vi "AutoFlex.vi"(0 "Inputs":T1={"Slider 1"=0.0, "Slider 2"=-0.007874015748031496}, 1 "Record":bool=TRUE, 2 "Save":bool=TRUE, 3 "Playback":bool, 5 "Delete":bool, 6 "Increase File ID":bool, 7 "Decrease File ID":bool) -> (20 "Outputs":T1={"Slider 1"=0.0, "Slider 2"=-0.007874015748031496}, 22 "File ID":i32)   [LabVIEW 2012]
uses:
  Joystick Event.ctl
panel:
  out "Info Path":path=path "C:/Users/FRC/Desktop/Autoflex/000.txt"
  out "Joystick Event":cluster{"Timestamp":u32, "Input":T1}={"Timestamp"=657367, "Input"={"Slider 1"=0.0, "Slider 2"=-0.007874015748031496}}
  out "Timestamp":u32=657367
  out "Joystick Event Array":cluster{"Timestamp":u32, "Input":T1}[](array[cluster])=[{"Timestamp"=234633, "Input"={"Slider 1"=-0.047244094488188976, "Slider 2"=0.0}}, {"Timestamp"=234778, "Input"={"Slider 1"=-0.08661417322834646, "Slider 2"=-0.06299212598425197}}, {"Timestamp"=234848, "Input"={"Slider 1"=-0.08661417322834646, "Slider 2"=-0.14173228346456693}}, {"Timestamp"=234900, "Input"={"Slider 1"=-0.10236220472440945, "Slider 2"=-0.18110236220472442}}, {"Timestamp"=234954, "Input"={"Slider 1"=-0.12598425196850394, "Slider 2"=-0.28346456692913385}}, {"Timestamp"=235026, "Input"={"Slider 1"=-0.12598425196850394, "Slider 2"=-0.3228346456692913}}, {"Timestamp"=235372, "Input"={"Slider 1"=-0.12598425196850394, "Slider 2"=-0.3464566929133858}}, {"Timestamp"=235433, "Input"={"Slider 1"=0.07874015748031496, "Slider 2"=-0.4015748031496063}}, {"Timestamp"=235492, "Input"={"Slider 1"=-0.16535433070866143, "Slider 2"=-0.44881889763779526}}, {"Timestamp"=235557, "Input"={"Slider 1"=-0.18110236220472442, "Slider 2"=-0.4881889763779528}}, {"Timestamp"=235623, "Input"={"Slider 1"=-0.18110236220472442, "Slider 2"=-0.5039370078740157}}, {"Timestamp"=236417, "Input"={"Slider 1"=-0.18110236220472442, "Slider 2"=-0.30708661417322836}}, {"Timestamp"=236495, "Input"={"Slider 1"=0.0, "Slider 2"=-0.023622047244094488}}, {"Timestamp"=236541, "Input"={"Slider 1"=0.0, "Slider 2"=-0.007874015748031496}}, {"Timestamp"=236695, "Input"={"Slider 1"=0.0, "Slider 2"=0.0}}, {"Timestamp"=236902, "Input"={"Slider 1"=0.0, "Slider 2"=0.031496062992125984}}, {"Timestamp"=236955, "Input"={"Slider 1"=0.03937007874015748, "Slider 2"=0.09448818897637795}}, {"Timestamp"=237014, "Input"={"Slider 1"=0.11811023622047244, "Slider 2"=0.1732283464566929}}, {"Timestamp"=237078, "Input"={"Slider 1"=0.023622047244094488, "Slider 2"=0.2755905511811024}}, {"Timestamp"=237136, "Input"={"Slider 1"=0.0, "Slider 2"=0.3543307086614173}}, {"Timestamp"=237217, "Input"={"Slider 1"=0.0, "Slider 2"=0.4566929133858268}}, {"Timestamp"=237272, "Input"={"Slider 1"=0.0, "Slider 2"=0.5196850393700787}}, {"Timestamp"=237332, "Input"={"Slider 1"=0.0, "Slider 2"=0.5433070866141733}}, {"Timestamp"=237398, "Input"={"Slider 1"=0.0, "Slider 2"=0.5590551181102362}}, {"Timestamp"=237460, "Input"={"Slider 1"=0.0, "Slider 2"=0.5826771653543307}}, {"Timestamp"=237774, "Input"={"Slider 1"=0.0, "Slider 2"=0.5039370078740157}}, {"Timestamp"=237798, "Input"={"Slider 1"=0.0, "Slider 2"=0.4566929133858268}}, {"Timestamp"=237854, "Input"={"Slider 1"=0.0, "Slider 2"=0.31496062992125984}}, {"Timestamp"=237914, "Input"={"Slider 1"=0.0, "Slider 2"=0.05511811023622047}}, {"Timestamp"=237973, "Input"={"Slider 1"=0.0, "Slider 2"=0.0}}, {"Timestamp"=238179, "Input"={"Slider 1"=-0.023622047244094488, "Slider 2"=0.0}}, {"Timestamp"=238417, "Input"={"Slider 1"=-0.047244094488188976, "Slider 2"=-0.007874015748031496}}, {"Timestamp"=238454, "Input"={"Slider 1"=-0.06299212598425197, "Slider 2"=-0.007874015748031496}}, {"Timestamp"=238577, "Input"={"Slider 1"=-0.06299212598425197, "Slider 2"=-0.047244094488188976}}, {"Timestamp"=238615, "Input"={"Slider 1"=-0.08661417322834646, "Slider 2"=-0.08661417322834646}}, {"Timestamp"=238761, "Input"={"Slider 1"=-0.10236220472440945, "Slider 2"=-0.3464566929133858}}, {"Timestamp"=238815, "Input"={"Slider 1"=-0.16535433070866143, "Slider 2"=-0.3858267716535433}}, {"Timestamp"=238937, "Input"={"Slider 1"=0.0, "Slider 2"=-0.4015748031496063}}, {"Timestamp"=238999, "Input"={"Slider 1"=-0.16535433070866143, "Slider 2"=-0.44881889763779526}}, {"Timestamp"=239062, "Input"={"Slider 1"=-0.16535433070866143, "Slider 2"=-0.4645669291338583}}, {"Timestamp"=239362, "Input"={"Slider 1"=-0.08661417322834646, "Slider 2"=-0.4645669291338583}}, {"Timestamp"=239439, "Input"={"Slider 1"=-0.08661417322834646, "Slider 2"=-0.3858267716535433}}, {"Timestamp"=239476, "Input"={"Slider 1"=-0.08661417322834646, "Slider 2"=-0.2677165354330709}}, {"Timestamp"=239513, "Input"={"Slider 1"=-0.06299212598425197, "Slider 2"=-0.16535433070866143}}, {"Timestamp"=239553, "Input"={"Slider 1"=-0.047244094488188976, "Slider 2"=-0.14173228346456693}}, {"Timestamp"=239592, "Input"={"Slider 1"=0.0, "Slider 2"=-0.08661417322834646}}, {"Timestamp"=239644, "Input"={"Slider 1"=0.0, "Slider 2"=-0.007874015748031496}}, {"Timestamp"=239722, "Input"={"Slider 1"=0.03937007874015748, "Slider 2"=-0.007874015748031496}}, {"Timestamp"=239757, "Input"={"Slider 1"=0.0, "Slider 2"=-0.007874015748031496}}, {"Timestamp"=489779, "Input"={"Slider 1"=-0.023622047244094488, "Slider 2"=-0.007874015748031496}}, {"Timestamp"=489877, "Input"={"Slider 1"=-0.023622047244094488, "Slider 2"=-0.03937007874015748}}, {"Timestamp"=489894, "Input"={"Slider 1"=-0.023622047244094488, "Slider 2"=-0.07086614173228346}}, {"Timestamp"=489919, "Input"={"Slider 1"=-0.03937007874015748, "Slider 2"=-0.11811023622047244}}, {"Timestamp"=489939, "Input"={"Slider 1"=-0.05511811023622047, "Slider 2"=-0.14960629921259844}}, {"Timestamp"=489980, "Input"={"Slider 1"=-0.07874015748031496, "Slider 2"=-0.25196850393700787}}, {"Timestamp"=490002, "Input"={"Slider 1"=-0.03937007874015748, "Slider 2"=-0.2992125984251969}}, {"Timestamp"=490038, "Input"={"Slider 1"=-0.03937007874015748, "Slider 2"=-0.3858267716535433}}, {"Timestamp"=490060, "Input"={"Slider 1"=-0.09448818897637795, "Slider 2"=-0.4015748031496063}}, {"Timestamp"=490099, "Input"={"Slider 1"=-0.14960629921259844, "Slider 2"=-0.4330708661417323}}, {"Timestamp"=490217, "Input"={"Slider 1"=-0.16535433070866143, "Slider 2"=-0.44881889763779526}}, {"Timestamp"=490237, "Input"={"Slider 1"=-0.16535433070866143, "Slider 2"=-0.4645669291338583}}, {"Timestamp"=490279, "Input"={"Slider 1"=-0.16535433070866143, "Slider 2"=-0.48031496062992124}}, {"Timestamp"=490317, "Input"={"Slider 1"=-0.16535433070866143, "Slider 2"=-0.49606299212598426}}, {"Timestamp"=490336, "Input"={"Slider 1"=-0.16535433070866143, "Slider 2"=-0.5118110236220472}}, {"Timestamp"=490357, "Input"={"Slider 1"=-0.16535433070866143, "Slider 2"=-0.5354330708661418}}, {"Timestamp"=490380, "Input"={"Slider 1"=-0.16535433070866143, "Slider 2"=-0.5511811023622047}}, {"Timestamp"=490419, "Input"={"Slider 1"=-0.1889763779527559, "Slider 2"=-0.5511811023622047}}, {"Timestamp"=490475, "Input"={"Slider 1"=-0.1889763779527559, "Slider 2"=-0.5669291338582677}}, {"Timestamp"=490498, "Input"={"Slider 1"=-0.2047244094488189, "Slider 2"=-0.5669291338582677}}, {"Timestamp"=490557, "Input"={"Slider 1"=-0.2204724409448819, "Slider 2"=-0.5669291338582677}}, {"Timestamp"=490739, "Input"={"Slider 1"=-0.2204724409448819, "Slider 2"=-0.4645669291338583}}, {"Timestamp"=490764, "Input"={"Slider 1"=-0.2204724409448819, "Slider 2"=-0.41732283464566927}}, {"Timestamp"=490785, "Input"={"Slider 1"=-0.2204724409448819, "Slider 2"=-0.3464566929133858}}, {"Timestamp"=490816, "Input"={"Slider 1"=-0.16535433070866143, "Slider 2"=-0.11811023622047244}}, {"Timestamp"=490839, "Input"={"Slider 1"=0.0, "Slider 2"=-0.03937007874015748}}, {"Timestamp"=490882, "Input"={"Slider 1"=0.0, "Slider 2"=-0.007874015748031496}}, {"Timestamp"=490934, "Input"={"Slider 1"=0.0, "Slider 2"=0.0}}, {"Timestamp"=490958, "Input"={"Slider 1"=0.15748031496062992, "Slider 2"=0.0}}, {"Timestamp"=490980, "Input"={"Slider 1"=0.0, "Slider 2"=0.0}}, {"Timestamp"=491056, "Input"={"Slider 1"=0.0, "Slider 2"=0.007874015748031496}}, {"Timestamp"=491122, "Input"={"Slider 1"=0.0, "Slider 2"=0.03937007874015748}}, {"Timestamp"=491143, "Input"={"Slider 1"=0.0, "Slider 2"=0.05511811023622047}}, {"Timestamp"=491175, "Input"={"Slider 1"=0.0, "Slider 2"=0.11811023622047244}}, {"Timestamp"=491196, "Input"={"Slider 1"=0.0, "Slider 2"=0.14960629921259844}}, {"Timestamp"=491217, "Input"={"Slider 1"=0.0, "Slider 2"=0.18110236220472442}}, {"Timestamp"=491237, "Input"={"Slider 1"=0.0, "Slider 2"=0.2125984251968504}}, {"Timestamp"=491262, "Input"={"Slider 1"=-0.05511811023622047, "Slider 2"=0.25196850393700787}}, {"Timestamp"=491297, "Input"={"Slider 1"=-0.07874015748031496, "Slider 2"=0.3937007874015748}}, {"Timestamp"=491332, "Input"={"Slider 1"=-0.09448818897637795, "Slider 2"=0.4251968503937008}}, {"Timestamp"=491355, "Input"={"Slider 1"=-0.09448818897637795, "Slider 2"=0.5196850393700787}}, {"Timestamp"=491416, "Input"={"Slider 1"=-0.03937007874015748, "Slider 2"=0.5196850393700787}}, {"Timestamp"=491496, "Input"={"Slider 1"=-0.09448818897637795, "Slider 2"=0.5196850393700787}}, {"Timestamp"=491598, "Input"={"Slider 1"=-0.11023622047244094, "Slider 2"=0.5196850393700787}}, {"Timestamp"=491657, "Input"={"Slider 1"=-0.14960629921259844, "Slider 2"=0.5196850393700787}}, {"Timestamp"=491717, "Input"={"Slider 1"=-0.16535433070866143, "Slider 2"=0.5196850393700787}}, {"Timestamp"=491858, "Input"={"Slider 1"=-0.11023622047244094, "Slider 2"=0.5196850393700787}}, {"Timestamp"=491894, "Input"={"Slider 1"=-0.09448818897637795, "Slider 2"=0.5196850393700787}}, {"Timestamp"=491943, "Input"={"Slider 1"=-0.07874015748031496, "Slider 2"=0.5196850393700787}}, {"Timestamp"=491977, "Input"={"Slider 1"=-0.05511811023622047, "Slider 2"=0.4094488188976378}}, {"Timestamp"=491996, "Input"={"Slider 1"=-0.05511811023622047, "Slider 2"=0.3937007874015748}}, {"Timestamp"=492036, "Input"={"Slider 1"=-0.05511811023622047, "Slider 2"=0.3464566929133858}}, {"Timestamp"=492058, "Input"={"Slider 1"=-0.05511811023622047, "Slider 2"=0.2992125984251969}}, {"Timestamp"=492082, "Input"={"Slider 1"=-0.03937007874015748, "Slider 2"=0.2677165354330709}}, {"Timestamp"=492116, "Input"={"Slider 1"=-0.03937007874015748, "Slider 2"=0.16535433070866143}}, {"Timestamp"=492178, "Input"={"Slider 1"=-0.09448818897637795, "Slider 2"=0.16535433070866143}}, {"Timestamp"=492481, "Input"={"Slider 1"=-0.09448818897637795, "Slider 2"=0.14960629921259844}}, {"Timestamp"=492495, "Input"={"Slider 1"=-0.09448818897637795, "Slider 2"=0.13385826771653545}}, {"Timestamp"=492519, "Input"={"Slider 1"=-0.09448818897637795, "Slider 2"=0.11811023622047244}}, {"Timestamp"=492540, "Input"={"Slider 1"=-0.09448818897637795, "Slider 2"=0.07086614173228346}}, {"Timestamp"=492574, "Input"={"Slider 1"=-0.03937007874015748, "Slider 2"=0.03937007874015748}}, {"Timestamp"=492623, "Input"={"Slider 1"=-0.03937007874015748, "Slider 2"=0.007874015748031496}}, {"Timestamp"=492666, "Input"={"Slider 1"=-0.023622047244094488, "Slider 2"=0.0}}, {"Timestamp"=492715, "Input"={"Slider 1"=0.0, "Slider 2"=0.0}}, {"Timestamp"=492736, "Input"={"Slider 1"=0.0, "Slider 2"=-0.007874015748031496}}, {"Timestamp"=492805, "Input"={"Slider 1"=-0.09448818897637795, "Slider 2"=-0.023622047244094488}}, {"Timestamp"=492836, "Input"={"Slider 1"=-0.09448818897637795, "Slider 2"=-0.10236220472440945}}, {"Timestamp"=492864, "Input"={"Slider 1"=-0.16535433070866143, "Slider 2"=-0.13385826771653545}}, {"Timestamp"=492898, "Input"={"Slider 1"=-0.2047244094488189, "Slider 2"=-0.2047244094488189}}, {"Timestamp"=492921, "Input"={"Slider 1"=-0.2204724409448819, "Slider 2"=-0.25196850393700787}}, {"Timestamp"=492937, "Input"={"Slider 1"=-0.2204724409448819, "Slider 2"=-0.2992125984251969}}, {"Timestamp"=492960, "Input"={"Slider 1"=-0.2204724409448819, "Slider 2"=-0.31496062992125984}}, {"Timestamp"=492996, "Input"={"Slider 1"=-0.2755905511811024, "Slider 2"=-0.33070866141732286}}, {"Timestamp"=493016, "Input"={"Slider 1"=-0.2992125984251969, "Slider 2"=-0.33070866141732286}}, {"Timestamp"=493079, "Input"={"Slider 1"=-0.2440944881889764, "Slider 2"=-0.33070866141732286}}, {"Timestamp"=493103, "Input"={"Slider 1"=-0.2047244094488189, "Slider 2"=-0.33070866141732286}}, {"Timestamp"=493118, "Input"={"Slider 1"=-0.2047244094488189, "Slider 2"=-0.2677165354330709}}, {"Timestamp"=493141, "Input"={"Slider 1"=-0.2047244094488189, "Slider 2"=-0.2204724409448819}}, {"Timestamp"=493175, "Input"={"Slider 1"=-0.1889763779527559, "Slider 2"=-0.14960629921259844}}, {"Timestamp"=493202, "Input"={"Slider 1"=-0.16535433070866143, "Slider 2"=-0.11811023622047244}}, {"Timestamp"=493238, "Input"={"Slider 1"=-0.09448818897637795, "Slider 2"=-0.03937007874015748}}, {"Timestamp"=493266, "Input"={"Slider 1"=-0.03937007874015748, "Slider 2"=-0.023622047244094488}}, {"Timestamp"=493300, "Input"={"Slider 1"=0.0, "Slider 2"=-0.007874015748031496}}, {"Timestamp"=493415, "Input"={"Slider 1"=-0.05511811023622047, "Slider 2"=-0.07086614173228346}}, {"Timestamp"=493442, "Input"={"Slider 1"=-0.05511811023622047, "Slider 2"=-0.11811023622047244}}, {"Timestamp"=493479, "Input"={"Slider 1"=-0.09448818897637795, "Slider 2"=-0.2677165354330709}}, {"Timestamp"=493498, "Input"={"Slider 1"=-0.09448818897637795, "Slider 2"=-0.4015748031496063}}, {"Timestamp"=493517, "Input"={"Slider 1"=-0.14960629921259844, "Slider 2"=-0.44881889763779526}}, {"Timestamp"=493543, "Input"={"Slider 1"=-0.1889763779527559, "Slider 2"=-0.48031496062992124}}, {"Timestamp"=493567, "Input"={"Slider 1"=-0.2204724409448819, "Slider 2"=-0.48031496062992124}}, {"Timestamp"=493698, "Input"={"Slider 1"=-0.16535433070866143, "Slider 2"=-0.48031496062992124}}, {"Timestamp"=493727, "Input"={"Slider 1"=-0.16535433070866143, "Slider 2"=-0.41732283464566927}}, {"Timestamp"=493754, "Input"={"Slider 1"=-0.16535433070866143, "Slider 2"=-0.33070866141732286}}, {"Timestamp"=493776, "Input"={"Slider 1"=-0.14960629921259844, "Slider 2"=-0.2047244094488189}}, {"Timestamp"=493795, "Input"={"Slider 1"=-0.13385826771653545, "Slider 2"=-0.11811023622047244}}, {"Timestamp"=493817, "Input"={"Slider 1"=-0.05511811023622047, "Slider 2"=-0.023622047244094488}}, {"Timestamp"=493836, "Input"={"Slider 1"=0.0, "Slider 2"=-0.007874015748031496}}, {"Timestamp"=494162, "Input"={"Slider 1"=0.0, "Slider 2"=0.0}}, {"Timestamp"=494184, "Input"={"Slider 1"=0.0, "Slider 2"=0.007874015748031496}}, {"Timestamp"=494224, "Input"={"Slider 1"=0.0, "Slider 2"=0.023622047244094488}}, {"Timestamp"=494238, "Input"={"Slider 1"=0.0, "Slider 2"=0.03937007874015748}}, {"Timestamp"=494277, "Input"={"Slider 1"=0.0, "Slider 2"=0.07086614173228346}}, {"Timestamp"=494299, "Input"={"Slider 1"=0.0, "Slider 2"=0.11811023622047244}}, {"Timestamp"=494337, "Input"={"Slider 1"=0.0, "Slider 2"=0.14960629921259844}}, {"Timestamp"=494361, "Input"={"Slider 1"=0.0, "Slider 2"=0.1968503937007874}}, {"Timestamp"=494400, "Input"={"Slider 1"=0.0, "Slider 2"=0.2992125984251969}}, {"Timestamp"=494416, "Input"={"Slider 1"=0.0, "Slider 2"=0.36220472440944884}}, {"Timestamp"=494439, "Input"={"Slider 1"=0.0, "Slider 2"=0.3937007874015748}}, {"Timestamp"=494458, "Input"={"Slider 1"=0.0, "Slider 2"=0.4251968503937008}}, {"Timestamp"=494476, "Input"={"Slider 1"=0.0, "Slider 2"=0.47244094488188976}}, {"Timestamp"=494502, "Input"={"Slider 1"=0.0, "Slider 2"=0.5039370078740157}}, {"Timestamp"=494543, "Input"={"Slider 1"=0.0, "Slider 2"=0.5196850393700787}}, {"Timestamp"=494578, "Input"={"Slider 1"=0.0, "Slider 2"=0.5354330708661418}}, {"Timestamp"=494613, "Input"={"Slider 1"=0.0, "Slider 2"=0.5511811023622047}}, {"Timestamp"=494647, "Input"={"Slider 1"=0.0, "Slider 2"=0.5669291338582677}}, {"Timestamp"=494737, "Input"={"Slider 1"=0.0, "Slider 2"=0.5039370078740157}}, {"Timestamp"=494776, "Input"={"Slider 1"=0.0, "Slider 2"=0.4409448818897638}}, {"Timestamp"=494798, "Input"={"Slider 1"=-0.03937007874015748, "Slider 2"=0.4409448818897638}}, {"Timestamp"=494835, "Input"={"Slider 1"=-0.07874015748031496, "Slider 2"=0.4094488188976378}}, {"Timestamp"=494856, "Input"={"Slider 1"=-0.09448818897637795, "Slider 2"=0.3937007874015748}}, {"Timestamp"=494896, "Input"={"Slider 1"=-0.09448818897637795, "Slider 2"=0.31496062992125984}}, {"Timestamp"=494918, "Input"={"Slider 1"=-0.03937007874015748, "Slider 2"=0.23622047244094488}}, {"Timestamp"=494937, "Input"={"Slider 1"=0.0, "Slider 2"=0.05511811023622047}}, {"Timestamp"=494961, "Input"={"Slider 1"=0.0, "Slider 2"=0.0}}, {"Timestamp"=494976, "Input"={"Slider 1"=0.0, "Slider 2"=-0.007874015748031496}}, {"Timestamp"=495102, "Input"={"Slider 1"=-0.05511811023622047, "Slider 2"=-0.007874015748031496}}, {"Timestamp"=495230, "Input"={"Slider 1"=-0.07874015748031496, "Slider 2"=-0.023622047244094488}}, {"Timestamp"=495256, "Input"={"Slider 1"=-0.07874015748031496, "Slider 2"=-0.10236220472440945}}, {"Timestamp"=495284, "Input"={"Slider 1"=-0.09448818897637795, "Slider 2"=-0.13385826771653545}}, {"Timestamp"=495334, "Input"={"Slider 1"=-0.13385826771653545, "Slider 2"=-0.25196850393700787}}, {"Timestamp"=495358, "Input"={"Slider 1"=-0.1889763779527559, "Slider 2"=-0.41732283464566927}}, {"Timestamp"=495400, "Input"={"Slider 1"=-0.2440944881889764, "Slider 2"=-0.5118110236220472}}, {"Timestamp"=495436, "Input"={"Slider 1"=-0.2992125984251969, "Slider 2"=-0.5669291338582677}}, {"Timestamp"=495459, "Input"={"Slider 1"=-0.2992125984251969, "Slider 2"=-0.6141732283464567}}, {"Timestamp"=495497, "Input"={"Slider 1"=-0.31496062992125984, "Slider 2"=-0.6614173228346457}}, {"Timestamp"=495519, "Input"={"Slider 1"=-0.31496062992125984, "Slider 2"=-0.6771653543307087}}, {"Timestamp"=495672, "Input"={"Slider 1"=-0.31496062992125984, "Slider 2"=-0.6141732283464567}}, {"Timestamp"=495694, "Input"={"Slider 1"=-0.31496062992125984, "Slider 2"=-0.5354330708661418}}, {"Timestamp"=495722, "Input"={"Slider 1"=-0.31496062992125984, "Slider 2"=-0.48031496062992124}}, {"Timestamp"=495759, "Input"={"Slider 1"=-0.2047244094488189, "Slider 2"=-0.25196850393700787}}, {"Timestamp"=495776, "Input"={"Slider 1"=-0.14960629921259844, "Slider 2"=-0.10236220472440945}}, {"Timestamp"=495817, "Input"={"Slider 1"=0.0, "Slider 2"=-0.007874015748031496}}, {"Timestamp"=495903, "Input"={"Slider 1"=0.0, "Slider 2"=0.0}}, {"Timestamp"=495998, "Input"={"Slider 1"=0.0, "Slider 2"=0.023622047244094488}}, {"Timestamp"=496022, "Input"={"Slider 1"=0.0, "Slider 2"=0.05511811023622047}}, {"Timestamp"=496076, "Input"={"Slider 1"=0.0, "Slider 2"=0.13385826771653545}}, {"Timestamp"=496100, "Input"={"Slider 1"=0.0, "Slider 2"=0.1968503937007874}}, {"Timestamp"=496141, "Input"={"Slider 1"=0.0, "Slider 2"=0.31496062992125984}}, {"Timestamp"=496181, "Input"={"Slider 1"=0.0, "Slider 2"=0.4094488188976378}}, {"Timestamp"=496227, "Input"={"Slider 1"=0.0, "Slider 2"=0.5196850393700787}}, {"Timestamp"=496556, "Input"={"Slider 1"=-0.05511811023622047, "Slider 2"=0.5196850393700787}}, {"Timestamp"=496598, "Input"={"Slider 1"=-0.05511811023622047, "Slider 2"=0.4409448818897638}}, {"Timestamp"=496615, "Input"={"Slider 1"=-0.05511811023622047, "Slider 2"=0.4094488188976378}}, {"Timestamp"=496635, "Input"={"Slider 1"=-0.05511811023622047, "Slider 2"=0.3779527559055118}}, {"Timestamp"=496657, "Input"={"Slider 1"=-0.05511811023622047, "Slider 2"=0.2992125984251969}}, {"Timestamp"=496696, "Input"={"Slider 1"=-0.05511811023622047, "Slider 2"=0.023622047244094488}}, {"Timestamp"=496716, "Input"={"Slider 1"=-0.05511811023622047, "Slider 2"=-0.007874015748031496}}, {"Timestamp"=653789, "Input"={"Slider 1"=0.0, "Slider 2"=-0.007874015748031496}}]
  out "Array size":i32=207
  out "Last Played Index":i32
  out "Retrieve Index":i32
  out "Start Time":u32
  out "File Path":path=path "C:/Users/FRC/Desktop/Autoflex/000.autoflex"
  out "Next Joystick Event":cluster{"Timestamp":u32, "Input":T1}
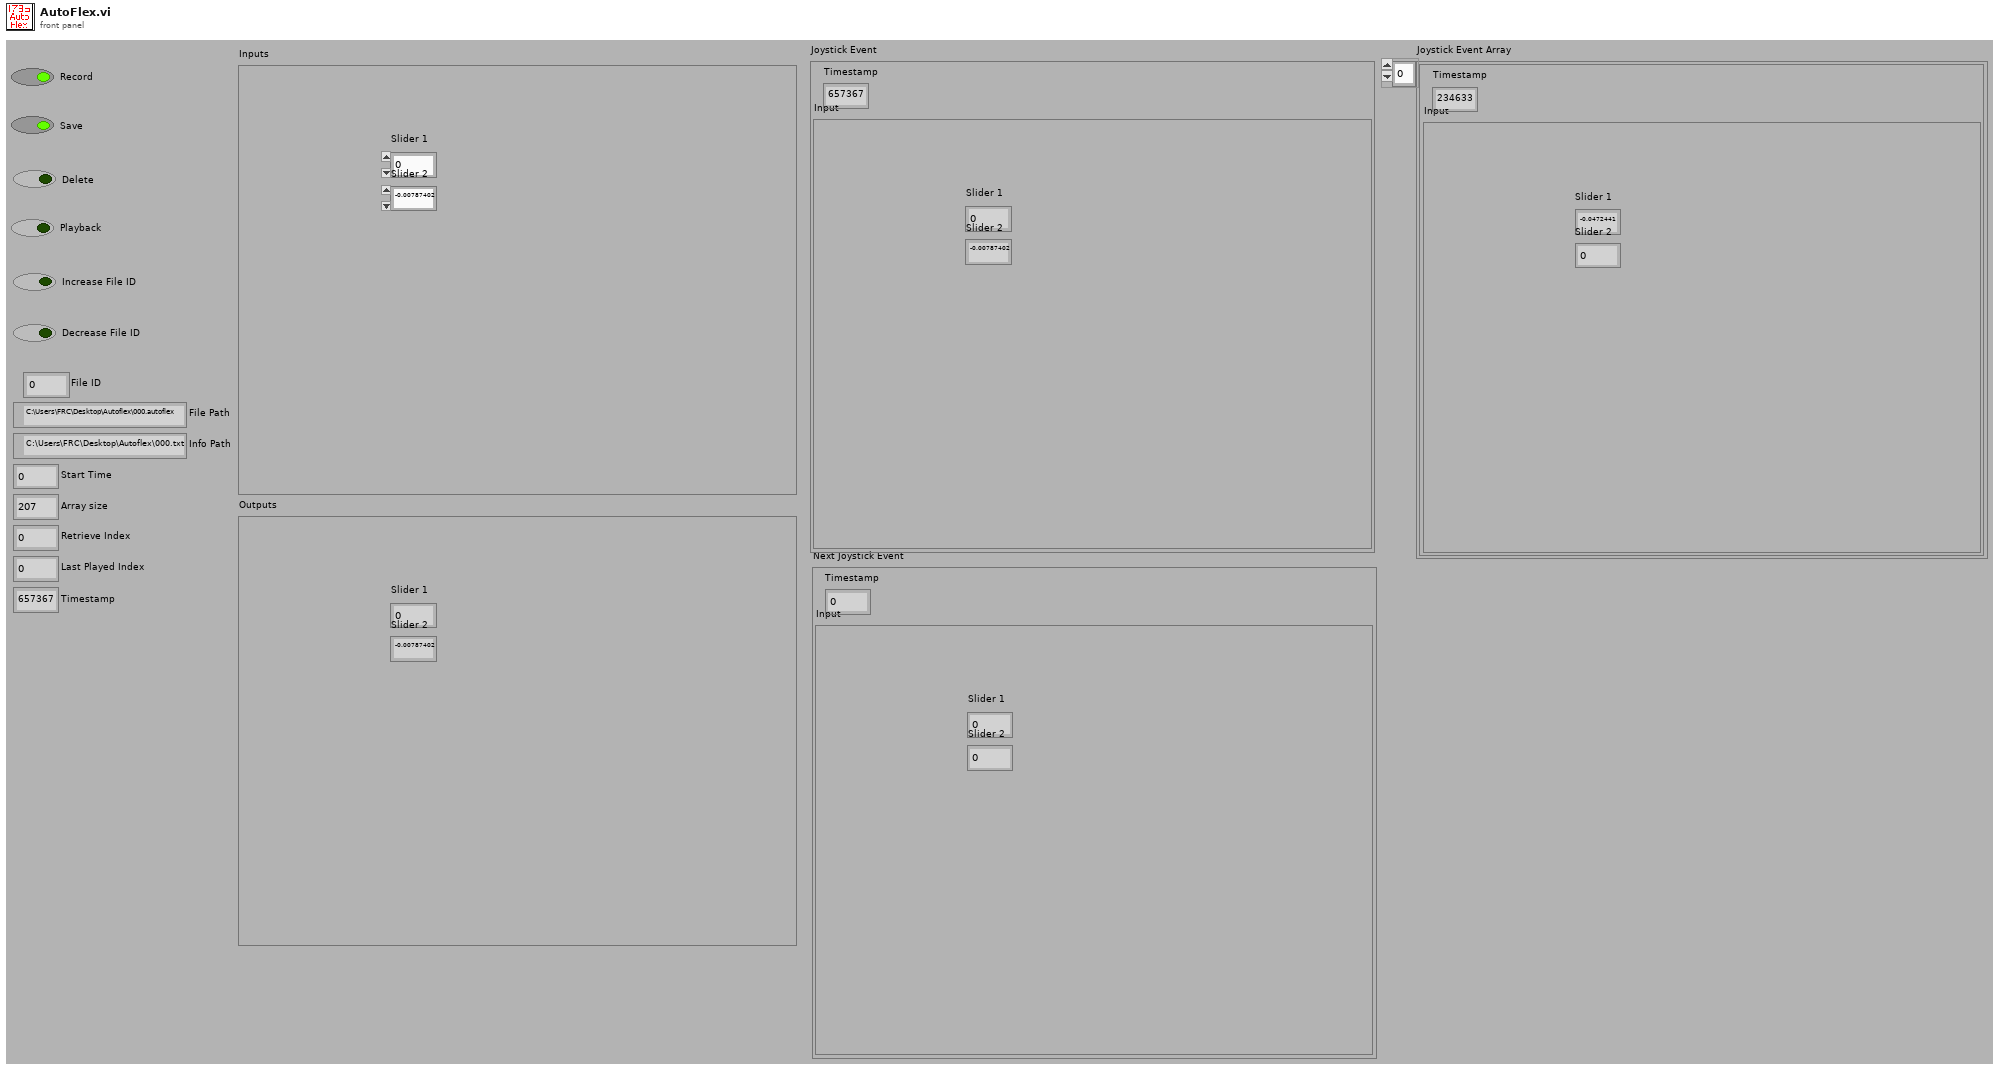
[diagram p1: front panel]
types:
  T1 = typedef "Joystick Event.ctl" = cluster{"Slider 1":dbl, "Slider 2":dbl}
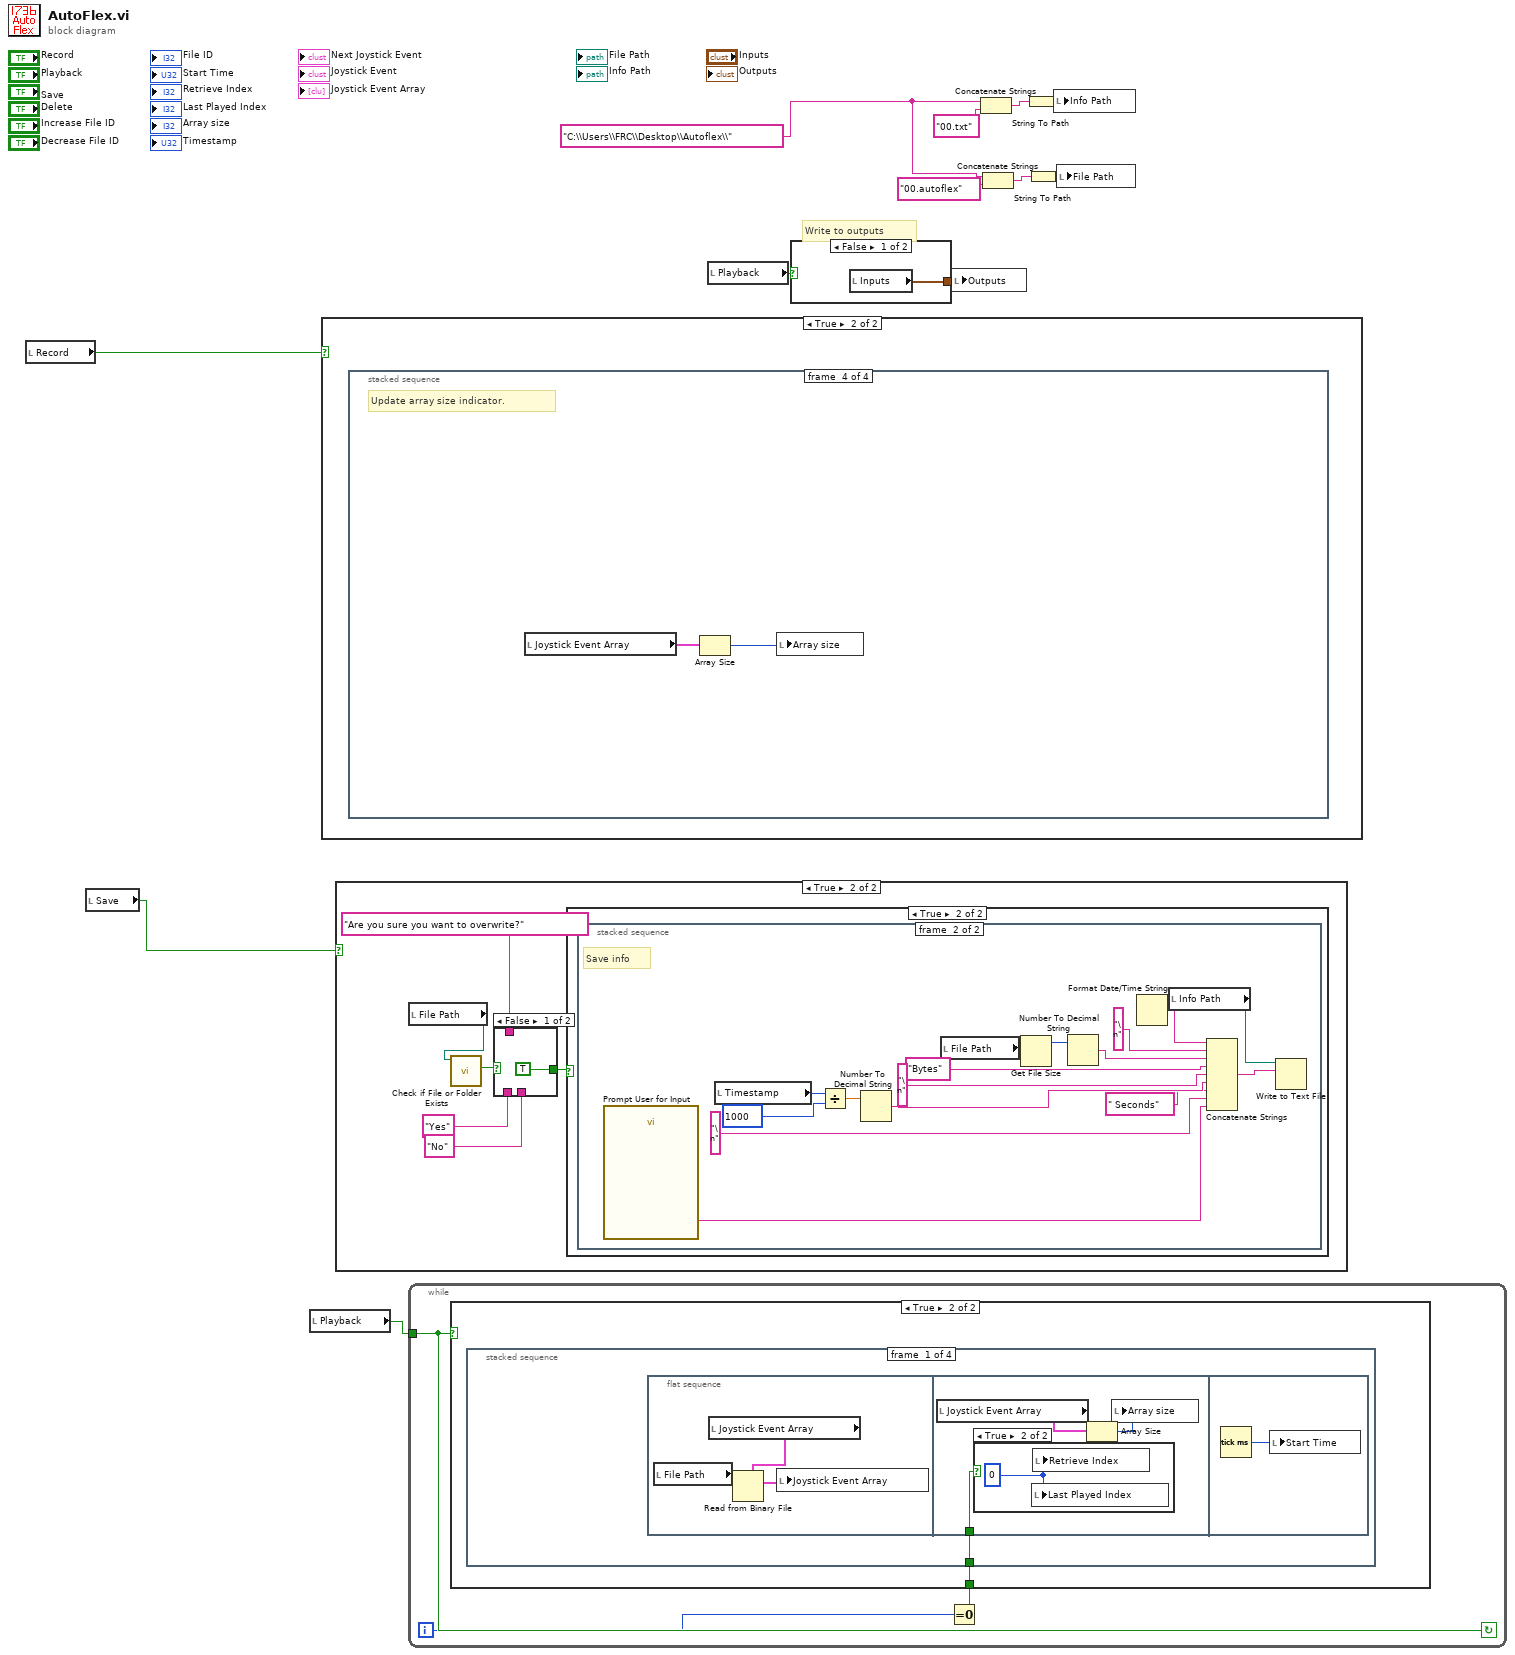
[diagram p0: block diagram]
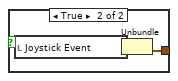
[diagram p2: hidden frame]
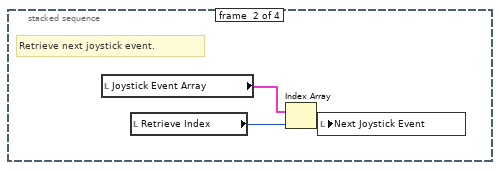
[diagram p5: hidden frame]
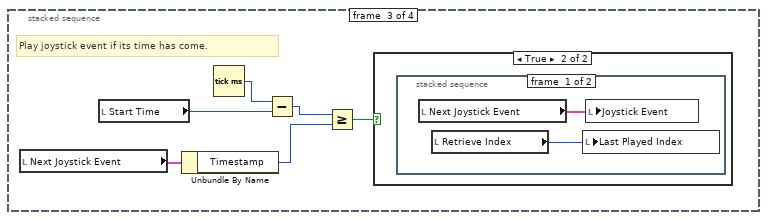
[diagram p6: hidden frame]
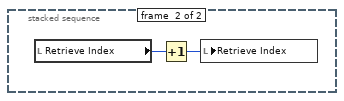
[diagram p8: hidden frame]
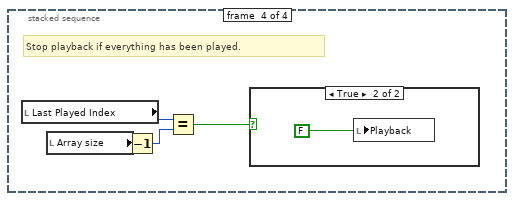
[diagram p9: hidden frame]
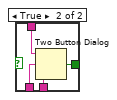
[diagram p12: hidden frame]
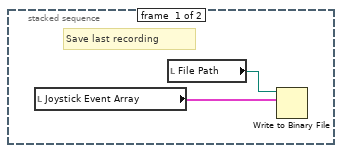
[diagram p14: hidden frame]
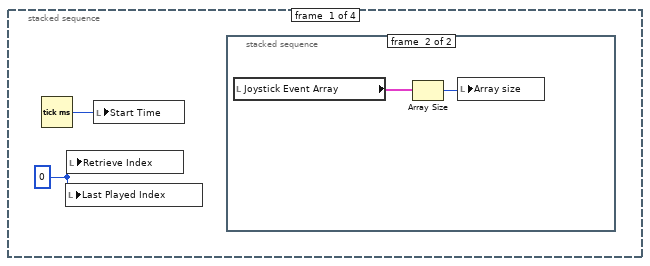
[diagram p16: hidden frame]
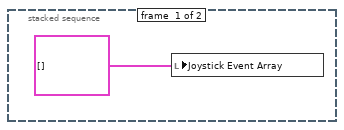
[diagram p17: hidden frame]
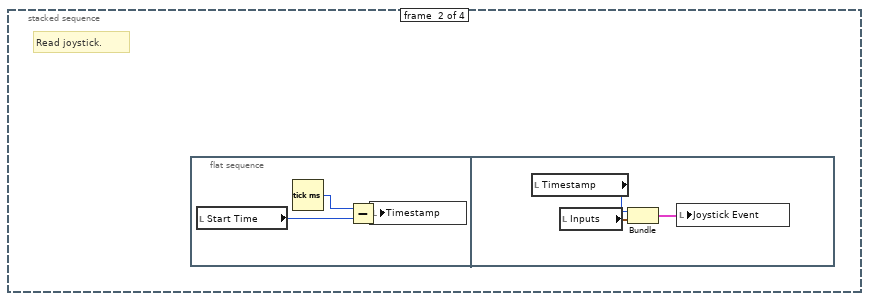
[diagram p18: hidden frame]
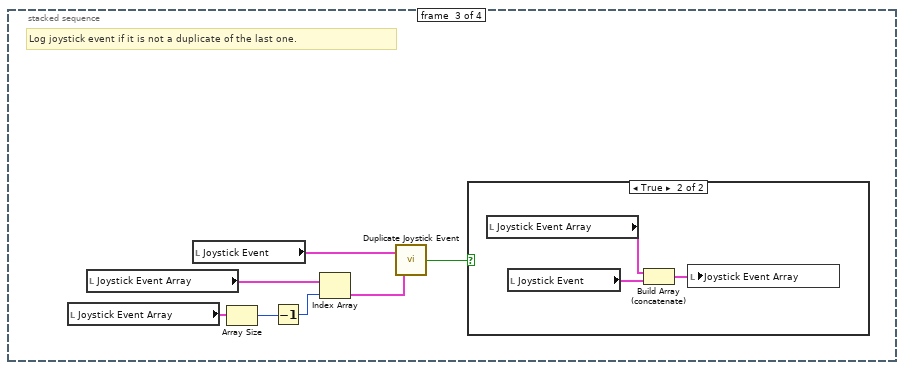
[diagram p19: hidden frame]
diagram:
  w3 = "C:\\Users\\FRC\\Desktop\\Autoflex\\" ("string")
  # "Write to outputs"
  n1 = local read "Record"() -> (w11:bool)
  n2 = local read "Save"() -> (w10:bool)
  n3 = local read "Playback"() -> (w12:bool)
  n4 = case shown="True" w11 {
    frame False {
    }
    frame True {
      n5 = stacked-sequence {
        frame #0 {
          w13 = 0 ("index")
          n6 = Tick Count (ms)() -> (millisecond timer value=w14:u32)
          n7 = local write "Last Played Index"(w13) -> ()
          n8 = local write "Retrieve Index"(w13) -> ()
          n9 = local write "Start Time"(w14) -> ()
          n10 = stacked-sequence {
            frame #0 {
              n11 = local write "Joystick Event Array"(cluster{"Timestamp":u32, "Input":T1}[] [] ("Joystick Event Array")) -> ()
            }
            frame #1 {
              n12 = local read "Joystick Event Array"() -> (w16:cluster{"Timestamp":u32, "Input":T1}[])
              n13 = Array Size(array=w16) -> (size(s)=w17:i32)
              n14 = local write "Array size"(w17) -> ()
            }
          }
        }
        frame #1 {
          # "Read joystick."
          n15 = flat-sequence {
            frame #0 {
              n16 = local read "Start Time"() -> (w19:u32)
              n17 = Tick Count (ms)() -> (millisecond timer value=w18:u32)
              n18 = Subtract(x=w18, y=w19) -> (x-y=w20:u32)
              n19 = local write "Timestamp"(w20) -> ()
            }
            frame #1 {
              n20 = local read "Timestamp"() -> (w22:u32)
              n21 = local read "Inputs"() -> (w21:T1)
              n22 = Bundle("Timestamp"=w22, "Inputs"=w21) -> (w23:cluster{"Timestamp":u32, "Inputs":T1})  [unwired: 1 out]
              n23 = local write "Joystick Event"(w23) -> ()
            }
          }
        }
        frame #2 {
          # "Log joystick event if it is not a duplicate of the last one."
          n24 = local read "Joystick Event Array"() -> (w28:cluster{"Timestamp":u32, "Input":T1}[])
          n25 = local read "Joystick Event Array"() -> (w27:cluster{"Timestamp":u32, "Input":T1}[])
          n26 = local read "Joystick Event"() -> (w25:cluster{"Timestamp":u32, "Input":T1})
          n27 = Array Size(array=w28) -> (size(s)=w30:i32)
          n28 = Decrement(x=w30) -> (x-1=w29:i32)
          n29 = Index Array(array=w27, index=w29) -> (element=w26:cluster{"Timestamp":u32, "Input":T1})
          n30 = call "Duplicate Joystick Event.vi"("Joystick Event 2"=w26, "Joystick Event 1"=w25) -> ("Duplicate"=w24:bool)
          n31 = case shown="True" w24 {
            frame False {
            }
            frame True {
              n32 = local read "Joystick Event Array"() -> (w31:cluster{"Timestamp":u32, "Input":T1}[])
              n33 = local read "Joystick Event"() -> (w33:cluster{"Timestamp":u32, "Input":T1})
              n34 = Build Array (concatenate)(w31, w33) -> (w32:cluster{"Timestamp":u32, "Input":T1}[])
              n35 = local write "Joystick Event Array"(w32) -> ()
            }
          }
        }
        frame #3 {
          # "Update array size indicator."
          n36 = local read "Joystick Event Array"() -> (w34:cluster{"Timestamp":u32, "Input":T1}[])
          n37 = Array Size(array=w34) -> (size(s)=w35:i32)
          n38 = local write "Array size"(w35) -> ()
        }
      }
    }
  }
  n39 = case shown="True" w10 {
    frame False {
    }
    frame True {
      n40 = local read "File Path"() -> (w39:path)
      n41 = call <vilib>:"Check if File or Folder Exists.vi"("path"=w39) -> ("file or folder exists?"=w40:bool)  [unwired: 1 in, 9 out]
      n42 = case shown="False" w40 {
        tunnel: [TRUE ("T button?") w46] -> w41
        tunnel: "Are you sure you want to overwrite?" ("message") -> [_ w45]
        tunnel: "Yes" ("T button name (\"OK\")") -> [_ w44]
        tunnel: "No" ("T button name (\"OK\")") -> [_ w43]
        frame False {
        }
        frame True {
          n43 = Two Button Dialog(message=w45, 1:w43, 2:w44) -> (T button?=w46:bool)
        }
      }
      n44 = case shown="True" w41 {
        frame False {
        }
        frame True {
          n45 = stacked-sequence {
            frame #0 {
              # "Save last recording"
              n46 = local read "Joystick Event Array"() -> (w47:cluster{"Timestamp":u32, "Input":T1}[])
              n47 = local read "File Path"() -> (w48:path)
              n48 = Write to Binary File(file (use dialog)=w48, data=w47) -> ()  [unwired: 1 in, 6 out]
            }
            frame #1 {
              # "Save info"
              n49 = call "Prompt User for Input"() -> ("Comments"=w50:string)  [unwired: 2 in, 17 out]
              n50 = local read "Timestamp"() -> (w55:u32)
              n51 = Divide(x=w55, y=u32 1000) -> (x/y=w52:dbl)
              n52 = Number To Decimal String(number=w52) -> (decimal integer string=w53:string)  [unwired: 1 out]
              n53 = local read "File Path"() -> (w64:path)
              n54 = Get File Size(file=w64) -> (size (in bytes)=w63:i64)  [unwired: 1 in, 2 out]
              n55 = Number To Decimal String(number=w63) -> (decimal integer string=w58:string)  [unwired: 1 out]
              n56 = Format Date/Time String() -> (date/time string=w60:string)  [unwired: 3 out]
              n57 = local read "Info Path"() -> (w62:path)
              n58 = Concatenate Strings(w60, "\n" ("string"), w58, "Bytes" ("string"), "\n" ("string"), w53, " Seconds" ("string"), "\n" ("string"), w50) -> (w61:string)
              n59 = Write to Text File(file (use dialog)=w62, text=w61) -> ()  [unwired: 1 in, 4 out]
            }
          }
        }
      }
    }
  }
  n60 = while {
    tunnel: w12 -> [w67]
    i -> [w66]
    stop <- w67 continue-if-true
    n61 = Equal To 0?(x=w66) -> (x = 0?=w65:bool)
    n62 = case shown="True" w67 {
      tunnel: w65 -> [_ w68]
      frame False {
      }
      frame True {
        n63 = stacked-sequence {
          tunnel: w68 -> [w69 _ _ _]
          frame #0 {
            n64 = flat-sequence {
              tunnel: w69 -> [w73]
              frame #0 {
                n65 = local read "File Path"() -> (w70:path)
                n66 = local read "Joystick Event Array"() -> (w71:cluster{"Timestamp":u32, "Input":T1}[])
                n67 = Read from Binary File(5:w71, 11:w70) -> (2:w72:cluster{"Timestamp":u32, "Input":T1}[])  [unwired: 1 in, 6 out]
                n68 = local write "Joystick Event Array"(w72) -> ()
              }
              frame #1 {
                n69 = local read "Joystick Event Array"() -> (w74:cluster{"Timestamp":u32, "Input":T1}[])
                n70 = case shown="True" w73 {
                  frame False {
                  }
                  frame True {
                    w76 = 0 ("index")
                    n71 = local write "Last Played Index"(w76) -> ()
                    n72 = local write "Retrieve Index"(w76) -> ()
                  }
                }
                n73 = Array Size(array=w74) -> (size(s)=w75:i32)
                n74 = local write "Array size"(w75) -> ()
              }
              frame #2 {
                n75 = Tick Count (ms)() -> (millisecond timer value=w77:u32)
                n76 = local write "Start Time"(w77) -> ()
              }
            }
          }
          frame #1 {
            # "Retrieve next joystick event."
            n77 = local read "Joystick Event Array"() -> (w79:cluster{"Timestamp":u32, "Input":T1}[])
            n78 = local read "Retrieve Index"() -> (w80:i32)
            n79 = Index Array(array=w79, index=w80) -> (element=w78:cluster{"Timestamp":u32, "Input":T1})
            n80 = local write "Next Joystick Event"(w78) -> ()
          }
          frame #2 {
            # "Play joystick event if its time has come."
            n81 = local read "Next Joystick Event"() -> (w84:cluster{"Timestamp":u32, "Input":T1})
            n82 = local read "Start Time"() -> (w81:u32)
            n83 = Unbundle By Name(w84) -> ("Timestamp"=w83:u32)
            n84 = Tick Count (ms)() -> (millisecond timer value=w82:u32)
            n85 = Subtract(x=w82, y=w81) -> (x-y=w85:u32)
            n86 = Greater Or Equal?(x=w85, y=w83) -> (x >= y?=w86:bool)
            n87 = case shown="True" w86 {
              frame False {
              }
              frame True {
                n88 = stacked-sequence {
                  frame #0 {
                    n89 = local read "Next Joystick Event"() -> (w87:cluster{"Timestamp":u32, "Input":T1})
                    n90 = local read "Retrieve Index"() -> (w88:i32)
                    n91 = local write "Last Played Index"(w88) -> ()
                    n92 = local write "Joystick Event"(w87) -> ()
                  }
                  frame #1 {
                    n93 = local read "Retrieve Index"() -> (w90:i32)
                    n94 = Increment(x=w90) -> (x+1=w89:i32)
                    n95 = local write "Retrieve Index"(w89) -> ()
                  }
                }
              }
            }
          }
          frame #3 {
            # "Stop playback if everything has been played."
            n96 = local read "Last Played Index"() -> (w91:i32)
            n97 = local read "Array size"() -> (w92:i32)
            n98 = Decrement(x=w92) -> (x-1=w94:i32)
            n99 = Equal?(x=w91, y=w94) -> (x = y?=w93:bool)
            n100 = case shown="True" w93 {
              frame False {
              }
              frame True {
                n101 = local write "Playback"(FALSE ("Playback Button")) -> ()
              }
            }
          }
        }
      }
    }
  }
  n102 = local read "Playback"() -> (w2:bool)
  n103 = case shown="False" w2 {
    tunnel: [w96 w97] -> w1
    frame False {
      n104 = local read "Inputs"() -> (w96:T1)
    }
    frame True {
      n105 = local read "Joystick Event"() -> (w98:cluster{"Timestamp":u32, "Input":T1})
      n106 = Unbundle(w98) -> ("Input"=w97:T1)  [unwired: 1 out]
    }
  }
  n107 = local write "Outputs"(w1) -> ()
  n108 = Concatenate Strings(w3, "00.txt" ("string")) -> (w5:string)
  n109 = Concatenate Strings(w3, "00.autoflex" ("string")) -> (w6:string)
  n110 = String To Path(string=w5) -> (path=w7:path)
  n111 = String To Path(string=w6) -> (path=w8:path)
  n112 = local write "Info Path"(w7) -> ()
  n113 = local write "File Path"(w8) -> ()
